vi "look_up_intensity.vi"(8 "error in (no error)":errorcluster, 10 "z offset":dbl[unit], 11 "depth/intensity points":T1) -> (0 "error out":errorcluster, 2 "intensity":dbl)   [LabVIEW 2010, in "XIntensityCompensation.xctl"]
uses:
  XIntensityCompensation.xctl
  data.ctl
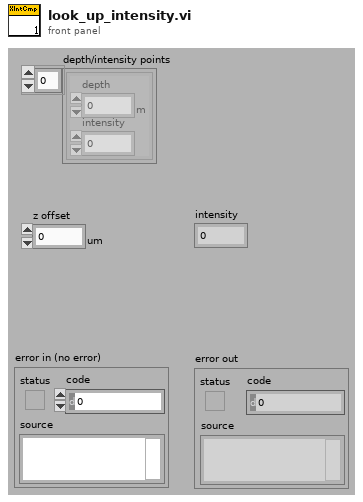
[diagram p1: front panel]
types:
  T1 = typedef "XIntensityCompensation.xctl/data.ctl" = cluster{"depth":dbl[unit], "intensity":dbl}[]
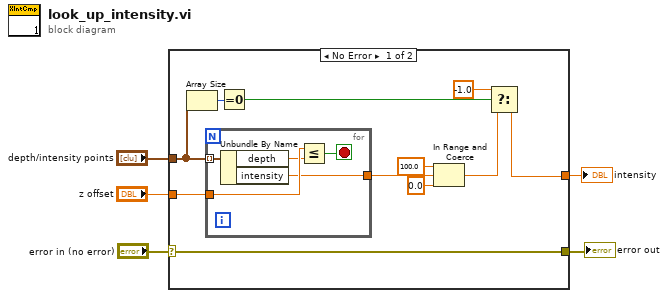
[diagram p0: block diagram]
diagram:
  n1 = case shown="No Error" "error in (no error)" {
    selector: "error in (no error)" -> [w15 w22]
    tunnel: "z offset" -> [w16 _]
    tunnel: "depth/intensity points" -> [w11 _]
    tunnel: [w15 w22] -> w2
    tunnel: [w6 _] -> w1
    frame No Error {
      n2 = Array Size(array=w11) -> (size(s)=w10:i32)
      n3 = for {
        tunnel: w11 -> [w21] mode=indexing
        tunnel: w16 -> [w20]
        tunnel: [w17] -> w14
        stop <- w18 stop-if-true
        n4 = Unbundle By Name(w21) -> ("depth"=w19:dbl[unit], "intensity"=w17:dbl)
        n5 = Less Or Equal?(x=w20, y=w19) -> (x <= y?=w18:bool)
      }
      n6 = Equal To 0?(x=w10) -> (x = 0?=w9:bool)
      n7 = In Range and Coerce(upper limit=100.0, x=w14, lower limit=0.0) -> (coerced(x)=w7:dbl)  [unwired: 1 out]
      n8 = Select(t=-1.0, s=w9, f=w7) -> (s? t:f=w6:dbl)
    }
    frame Error {
    }
  }
  "error out" <- w2
  "intensity" <- w1
